vi "Update Graph Properties.vi"(6 "Plot Ages":string, 7 "Timeout?":bool, 8 "error in (no error)":errorcluster, 9 "Current Data":T1 caption="All Data Cluster", 11 "Waveform Refs":refnum<vi>[](array[refnum])) -> (0 "error out":errorcluster)   [LabVIEW 2018, in "Testing UI 3.lvlib"]
uses:
  Testing UI 3.lvlib
  Top Level/Shared Controls/All Data Cluster.ctl
  Top Level/Shared Controls/Acq Data.ctl
  Top Level/Shared Controls/Post-Analysis Data.ctl
  Top Level/Shared Controls/Calculated Data.ctl
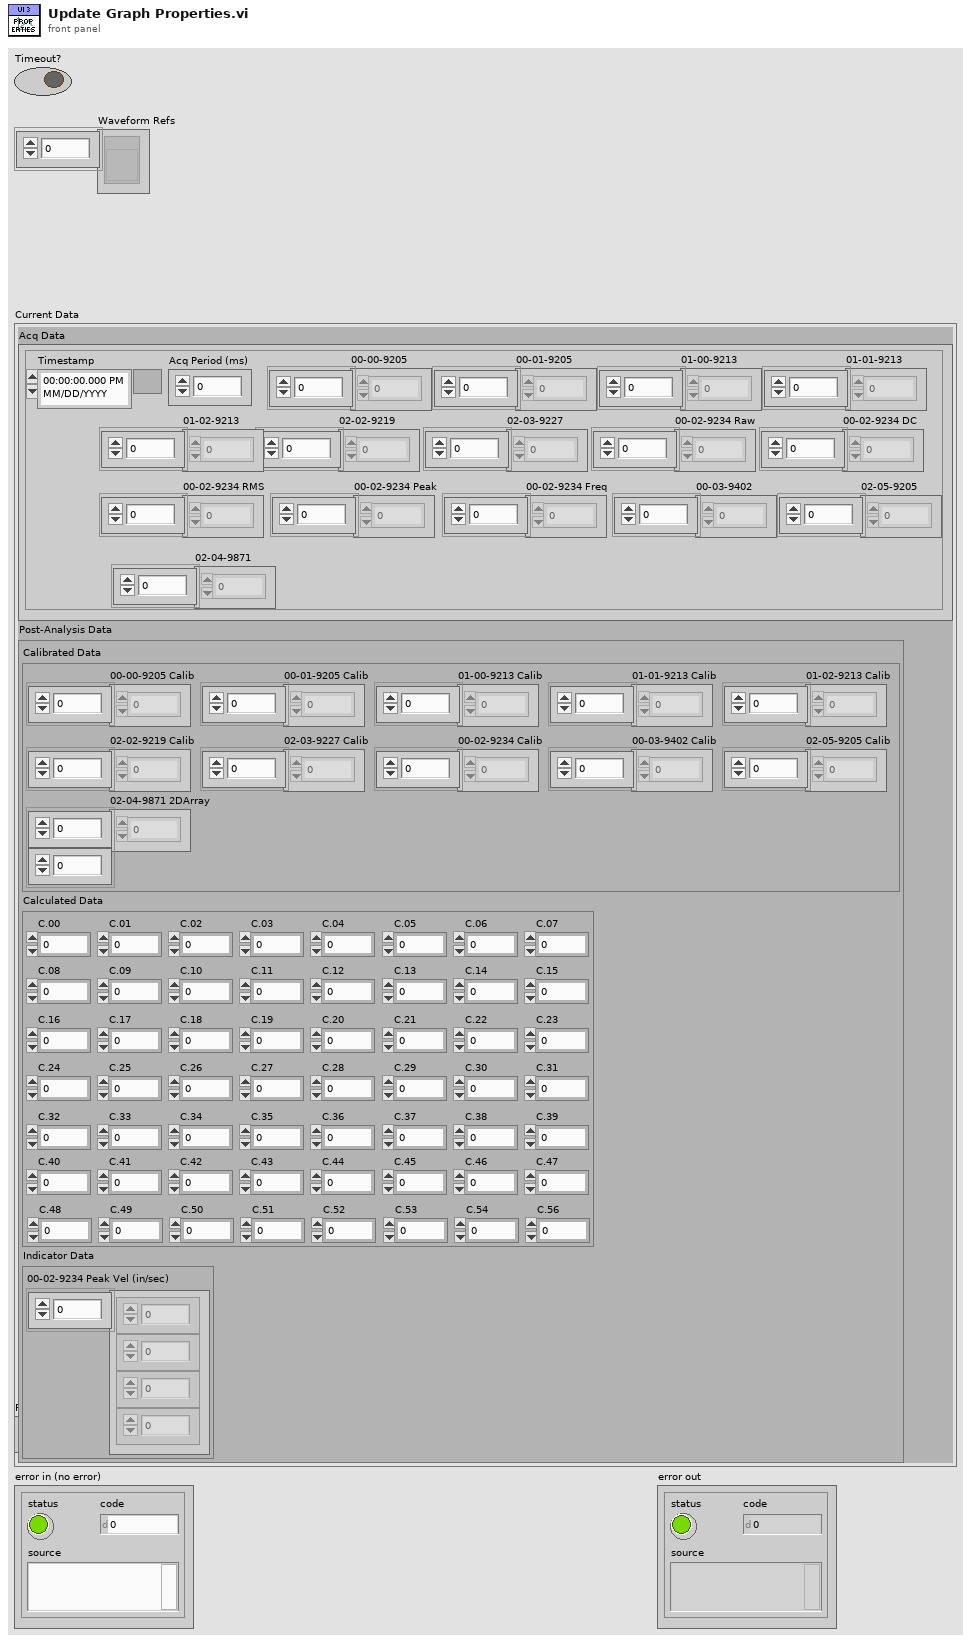
[diagram p1: front panel]
types:
  T1 = typedef "All Data Cluster.ctl" = cluster{"Acq Data":T2, "Post-Analysis Data":T3}
  T2 = typedef "Acq Data.ctl" = cluster{"Timestamp":timestamp, "Acq Period (ms)":i64, "00-00-9205":dbl[], "00-01-9205":dbl[], "01-00-9213":dbl[], "01-01-9213":dbl[], "01-02-9213":dbl[], "02-02-9219":dbl[], "02-03-9227":dbl[], "00-02-9234 Raw":dbl[], "00-02-9234 DC":dbl[], "00-02-9234 RMS":dbl[], "00-02-9234 Peak":dbl[], "00-02-9234 Freq":dbl[], "00-03-9402":dbl[], "02-05-9205":dbl[], "02-04-9871":dbl[]}
  T3 = typedef "Post-Analysis Data.ctl" = cluster{"Calibrated Data":cluster{"00-00-9205 Calib":dbl[], "00-01-9205 Calib":dbl[], "01-00-9213 Calib":dbl[], "01-01-9213 Calib":dbl[], "01-02-9213 Calib":dbl[], "02-02-9219 Calib":dbl[], "02-03-9227 Calib":dbl[], "00-02-9234 Calib":dbl[], "00-03-9402 Calib":dbl[], "02-05-9205 Calib":dbl[], "02-04-9871 2DArray":dbl[][]}, "Calculated Data":T4, "Indicator Data":cluster{"00-02-9234 Peak Vel (in/sec)":dbl[]}}
  T4 = typedef "Calculated Data.ctl" = cluster{"C.00":dbl, "C.01":dbl, "C.02":dbl, "C.03":dbl, "C.04":dbl, "C.05":dbl, "C.06":dbl, "C.07":dbl, "C.08":dbl, "C.09":dbl, "C.10":dbl, "C.11":dbl, "C.12":dbl, "C.13":dbl, "C.14":dbl, "C.15":dbl, "C.16":dbl, "C.17":dbl, "C.18":dbl, "C.19":dbl, "C.20":dbl, "C.21":dbl, "C.22":dbl, "C.23":dbl, "C.24":dbl, "C.25":dbl, "C.26":dbl, "C.27":dbl, "C.28":dbl, "C.29":dbl, "C.30":dbl, "C.31":dbl, "C.32":dbl, "C.33":dbl, "C.34":dbl, "C.35":dbl, "C.36":dbl, "C.37":dbl, "C.38":dbl, "C.39":dbl, "C.40":dbl, "C.41":dbl, "C.42":dbl, "C.43":dbl, "C.44":dbl, "C.45":dbl, "C.46":dbl, "C.47":dbl, "C.48":dbl, "C.49":dbl, "C.50":dbl, "C.51":dbl, "C.52":dbl, "C.53":dbl, "C.54":dbl, "C.56":dbl}
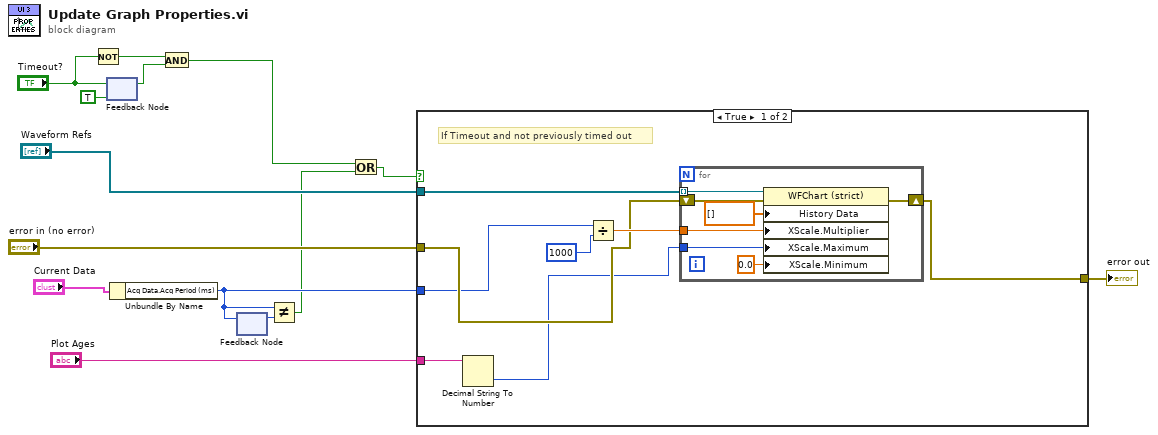
[diagram p0: block diagram]
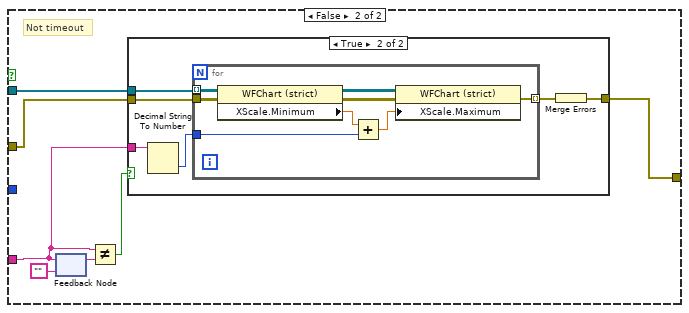
[diagram p2: hidden frame]
diagram:
  n1 = Not(x="Timeout?") -> (.not. x?=w11:bool)
  n2 = feedback #1(TRUE) -> (w9:bool)
  n3 = feedback-in #1("Timeout?") -> ()
  n4 = Unbundle By Name("Current Data") -> ("Acq Data.Acq Period (ms)"=w3:i64)
  n5 = And(x=w11, y=w9) -> (x .and. y?=w6:bool)
  n6 = feedback-in #2(w3) -> ()
  n7 = feedback #2() -> (w4:i64)  [unwired: 1 in]
  n8 = Not Equal?(x=w3, y=w4) -> (x != y?=w2:bool)
  n9 = Or(x=w6, y=w2) -> (x .or. y?=w5:bool)
  n10 = case shown="True" w5 {
    tunnel: "Waveform Refs" -> [w22 w33]
    tunnel: "error in (no error)" -> [w18 w32]
    tunnel: [w21 w31] -> w1
    tunnel: "Plot Ages" -> [w17 w30]
    tunnel: w3 -> [w15 _]
    frame True {
      # "If Timeout and not previously timed out"
      n11 = Decimal String To Number(string=w17) -> (number=w16:i32)  [unwired: 2 in, 1 out]
      n12 = Divide(x=w15, y=i64 1000) -> (x/y=w19:dbl)
      n13 = for {
        tunnel: w22 -> [w29] mode=indexing
        tunnel: w19 -> [w27]
        tunnel: w16 -> [w23]
        shift-right: [w26] -> w21
        shift-left: w18 -> [w28]
        n14 = property class="WFChart (strict)"(reference=w29, error in=w28, "History Data"=dbl[] [], "XScale.Multiplier"=w27, "XScale.Maximum"=w23, "XScale.Minimum"=0.0 ("X Scale.Range:Minimum")) -> (error out=w26:errorcluster)  [unwired: 1 out]
      }
    }
    frame False {
      # "Not timeout"
      n15 = feedback #3("" ("Plot Ages")) -> (w36:string)
      n16 = feedback-in #3(w30) -> ()
      n17 = Not Equal?(x=w30, y=w36) -> (x != y?=w34:bool)
      n18 = case shown="True" w34 {
        tunnel: w32 -> [w37 w41]
        tunnel: w33 -> [_ w42]
        tunnel: w30 -> [_ w43]
        tunnel: [w37 w38] -> w31
        frame False {
        }
        frame True {
          n19 = Decimal String To Number(string=w43) -> (number=w40:i32)  [unwired: 2 in, 1 out]
          n20 = for {
            tunnel: w42 -> [w50] mode=indexing
            tunnel: w41 -> [w49]
            tunnel: [w51] -> w39 mode=indexing
            tunnel: w40 -> [w45]
            n21 = property class="WFChart (strict)"(reference=w50, error in=w49) -> (reference out=w48:refnum<vi>, error out=w47:errorcluster, "XScale.Minimum"=w46:dbl)
            n22 = Add(x=w46, y=w45) -> (x+y=w44:dbl)
            n23 = property class="WFChart (strict)"(reference=w48, error in=w47, "XScale.Maximum"=w44) -> (error out=w51:errorcluster)  [unwired: 1 out]
          }
          n24 = Merge Errors(w39) -> (w38:errorcluster)
        }
      }
    }
  }
  "error out" <- w1
